vi "TDMS Example.vi"() -> ()   [LabVIEW 2020]
uses:
  Source/TDMS/TDMS Sink.lvclass
  C:/Users/hughe_cx/Documents/LVLog/Source/Sink/Sink.lvclass
  Source/LV Log.lvlib
  Source/Type Defs/Debug Level.ctl
panel:
  in  "Log Path":path
  in  "error in (no error)":errorcluster
  in  "Debug Level":T1=enum."DEBUG"
  out "error out":errorcluster
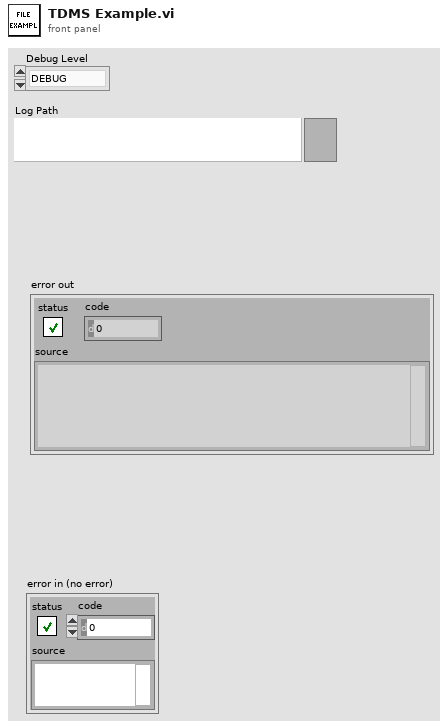
[diagram p1: front panel]
types:
  T1 = typedef "LV Log.lvlib/Debug Level.ctl" = enum16{"DEFAULT", "DEBUG", "INFO", "WARN", "ERROR", "FATAL"}
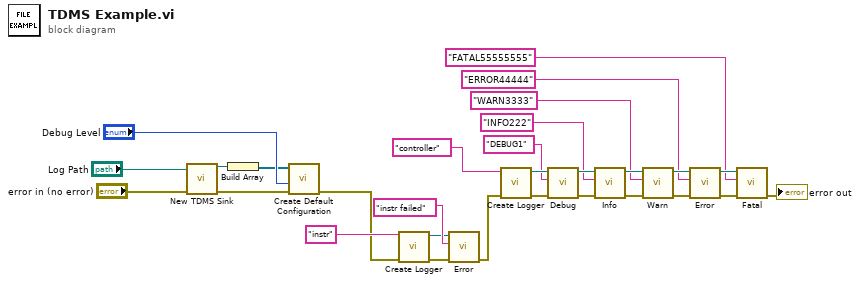
[diagram p0: block diagram]
diagram:
  n1 = call "New TDMS Sink.vi"("error in (no error)"="error in (no error)", "TDMS File Path"="Log Path") -> ("error out"=w6:errorcluster, "TDMS out"=w2:refnum<class "TDMS Sink.lvclass">)  [unwired: 8 in]
  n2 = Build Array(w2) -> (w1:refnum<class "TDMS Sink.lvclass">[])
  n3 = call "Create Default Configuration.vi"("Sinks"=w1, "Debug Level in"="Debug Level", "error in (no error)"=w6) -> ("error out"=w7:errorcluster)  [unwired: 7 in]
  n4 = call "Create Logger.vi"("error in (no error)"=w7, "Name"="instr") -> ("error out"=w9:errorcluster, "Logger out"=w10:refnum<class "Logger.lvclass">)  [unwired: 8 in]
  n5 = call "Error.vi"("error in (no error)"=w9, "Log Text"="instr failed", "Logger in"=w10) -> ("error out"=w11:errorcluster)  [unwired: 7 in, 1 out]
  n6 = call "Create Logger.vi"("error in (no error)"=w11, "Name"="controller") -> ("error out"=w28:errorcluster, "Logger out"=w27:refnum<class "Logger.lvclass">)  [unwired: 8 in]
  n7 = call "Debug.vi"("error in (no error)"=w28, "Log Text"="DEBUG1", "Logger in"=w27) -> ("error out"=w25:errorcluster, "Logger out"=w26:refnum<class "Logger.lvclass">)  [unwired: 7 in]
  n8 = call "Info.vi"("error in (no error)"=w25, "Log Text"="INFO222", "Logger in"=w26) -> ("error out"=w24:errorcluster, "Logger out"=w23:refnum<class "Logger.lvclass">)  [unwired: 7 in]
  n9 = call "Warn.vi"("error in (no error)"=w24, "Log Text"="WARN3333", "Logger in"=w23) -> ("error out"=w21:errorcluster, "Logger out"=w22:refnum<class "Logger.lvclass">)  [unwired: 7 in]
  n10 = call "Error.vi"("error in (no error)"=w21, "Log Text"="ERROR44444", "Logger in"=w22) -> ("error out"=w20:errorcluster, "Logger out"=w19:refnum<class "Logger.lvclass">)  [unwired: 7 in]
  n11 = call "Fatal.vi"("error in (no error)"=w20, "Log Text"="FATAL55555555", "Logger in"=w19) -> ("error out"=→"error out":errorcluster)  [unwired: 7 in, 1 out]
